vi "Load Device Database Into Cluster.vi"(8 "error in":errorcluster, 9 "system db":T1, 10 "cluster name (CAN0)":string="CAN0", 11 "database in":refnum<k21>=":memory:") -> (0 "error out":errorcluster, 2 "cluster out":refnum<k21>, 3 "database out":refnum<k21>)   [LabVIEW 2013, in "J1939.lvlib"]
uses:
  TypeDefs/J1939 db.ctl
  TypeDefs/J1939 db frame.ctl
  TypeDefs/J1939 db signal.ctl
  <vilib>/xnet/xnet.llb/XNET Database Create (Cluster).vi
  J1939.lvlib
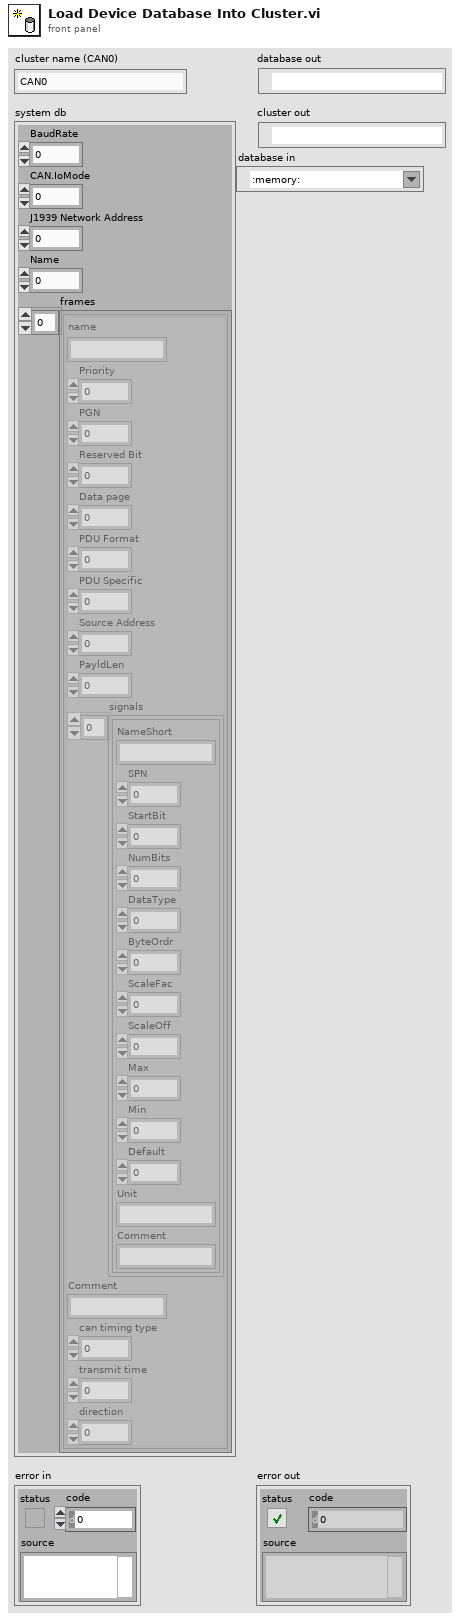
[diagram p1: front panel]
types:
  T1 = typedef "J1939.lvlib/J1939 db.ctl" = cluster{"BaudRate":u32, "CAN.IoMode":u32, "J1939 Network Address":u8, "Name":u64, "frames":T2[]}
  T2 = typedef "J1939.lvlib/J1939 db frame.ctl" = cluster{"name":string, "Priority":u8, "PGN":u32, "Reserved Bit":u8, "Data page":u8, "PDU Format":u8, "PDU Specific":u8, "Source Address":u8, "PayldLen":u32, "signals":T3[], "Comment":string, "can timing type":u32, "transmit time":dbl, "direction":u16}
  T3 = typedef "J1939.lvlib/J1939 db signal.ctl" = cluster{"NameShort":string, "SPN":i32, "StartBit":u32, "NumBits":u32, "DataType":u32, "ByteOrdr":u32, "ScaleFac":dbl, "ScaleOff":dbl, "Max":dbl, "Min":dbl, "Default":dbl, "Unit":string, "Comment":string}
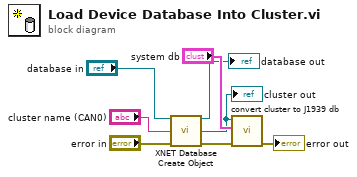
[diagram p0: block diagram]
diagram:
  n1 = call-poly <vilib>:"XNET Database Create Object.vi"("database in"="database in", "cluster name"="cluster name (CAN0)", "error in (no error)"="error in") -> ("database out"=→"database out":refnum<k21>, "cluster out"=w3:refnum<k21>, "error out"=w6:errorcluster)  [unwired: 10 in]
  "cluster out" <- w3
  n2 = call "convert cluster to J1939 db.vi"("error in"=w6, "system db"="system db", "db cluster"=w3) -> ("error out"=→"error out":errorcluster)  [unwired: 8 in]
